vi "exitcom.vi"(8 "error in (no error)":errorcluster, 11 "MSCU":refnum<class "MSCU.lvclass">) -> (0 "error out":errorcluster, 2 "Status":string, 3 "MSCU":refnum<class "MSCU.lvclass">)   [LabVIEW 2019, in "MSCU.lvclass"]
uses:
  MSCU.lvclass
  MSCU.lvclass/MSCU.ctl
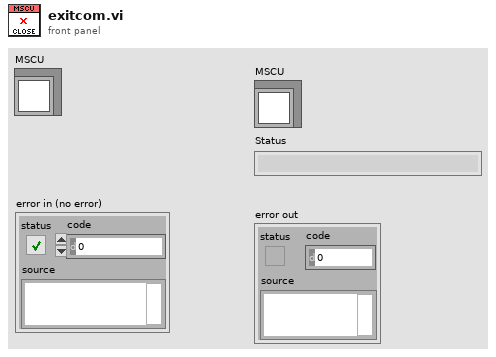
[diagram p1: front panel]
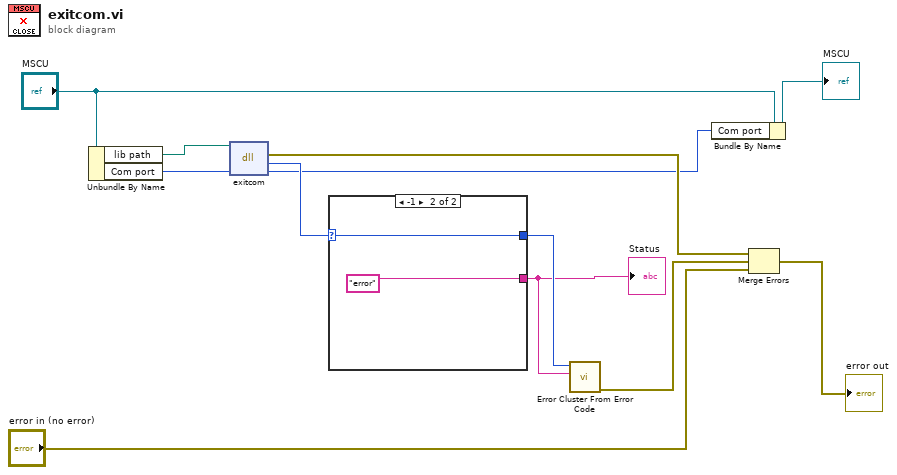
[diagram p0: block diagram]
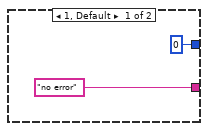
[diagram p2: hidden frame]
diagram:
  n1 = Unbundle By Name("MSCU") -> ("lib path"=w1:path, "Com port"=w5:i32)
  n2 = dll-call lib="C:/Program Files (x86)/Nanonis/SPM Controller/data/MSCU.dll" fn="exitcom"(path in=w1, "Comport"=w5) -> (error out=w9:errorcluster, "return type"=w12:i32, "Comport"=w6:i32)  [unwired: 2 in, 1 out]
  n3 = case shown="-1" w12 {
    selector: w12 -> [_ w16]
    tunnel: ["no error" "error"] -> w10
    tunnel: [0 ("return type") w16] -> w11
    frame 1, Default {
    }
    frame -1 {
    }
  }
  "Status" <- w10
  n4 = call <vilib>:"Error Cluster From Error Code.vi"("error message (\"\")"=w10, "error code (0)"=w11) -> ("error out"=w8:errorcluster)  [unwired: 7 in]
  n5 = Bundle By Name(cluster="MSCU", "Com port"=w6) -> (→"MSCU":refnum<class "MSCU.lvclass">)
  n6 = Merge Errors(w9, w8, "error in (no error)") -> (→"error out":errorcluster)
